vi "myRIO v1.0 Block Write Configuration.vi"() -> ()   [LabVIEW 2021]
panel:
  in  "Max Buffer Depth":u32=5
  in  "Max Samples":u32=10000
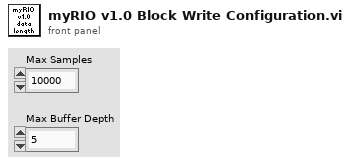
[diagram p1: front panel]
diagram:
